vi "Close_Popup.vi"(0 "Reference_In":refnum<vi>, 11 "Error_In":errorcluster) -> (4 "Reference_Out":refnum<vi>, 15 "Error_Out":errorcluster)   [LabVIEW 2021]
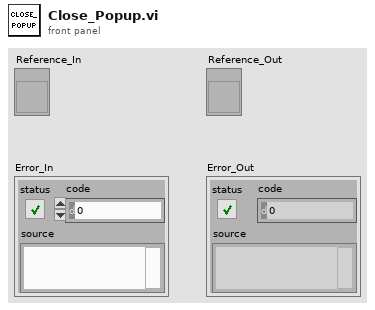
[diagram p1: front panel]
types:
  T1 = enum32{"Bad", "Idle", "Run top level", "Running"}
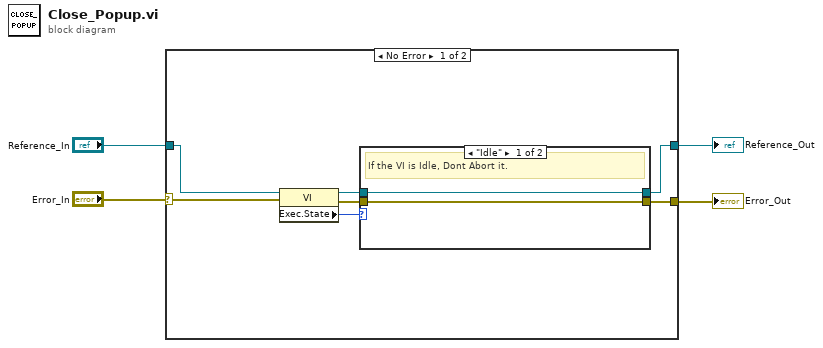
[diagram p0: block diagram]
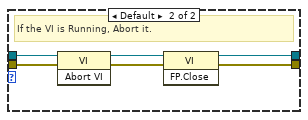
[diagram p2: hidden frame]
diagram:
  n1 = case shown="No Error" "Error_In" {
    selector: "Error_In" -> [w5 w20]
    tunnel: "Reference_In" -> [w8 w21]
    tunnel: [w7 w20] -> w3
    tunnel: [w6 w21] -> w2
    frame No Error {
      n2 = property on="Property Node" class="VI"(reference=w8, error in=w5) -> (reference out=w11:refnum<vi>, error out=w10:errorcluster, "Exec.State"=w9:T1)
      n3 = case shown="\"Idle\"" w9 {
        tunnel: w11 -> [w13 w19]
        tunnel: w10 -> [w12 w18]
        tunnel: [w13 w15] -> w6
        tunnel: [w12 w14] -> w7
        frame "Idle" {
          # "If the VI is Idle, Dont Abort it."
        }
        frame Default {
          # "If the VI is Running, Abort it."
          n4 = invoke on="Invoke Node" class="VI" method="Abort VI"(reference=w19, error in=w18) -> (reference out=w17:refnum<vi>, error out=w16:errorcluster)  [unwired: 1 in, 1 out]
          n5 = invoke class="VI" method="FP.Close"(reference=w17, error in=w16) -> (reference out=w15:refnum<vi>, error out=w14:errorcluster)  [unwired: 1 in, 1 out]
        }
      }
    }
    frame Error {
    }
  }
  "Reference_Out" <- w2
  "Error_Out" <- w3
